vi "test Quadrature.vi"(8 "error in (no error)":errorcluster, 11 "TestCase in":refnum<class "Scan Engine cRIO System Tests.lvclass">) -> (0 "error out":errorcluster, 3 "TestCase out":refnum<class "Scan Engine cRIO System Tests.lvclass">)   [LabVIEW 2016, in "Scan Engine cRIO System Tests.lvclass"]
uses:
  Scan Engine cRIO System Tests.lvclass
  C:/Users/rzoeller/Documents/ni-official/niveristand-custom-device-testing-tools/VeriStandTestCase/VeriStandTestCase.lvclass
  <vilib>/NI Veristand/Execution/Workspace/NI VeriStand - Get Single Channel Value.vi
  <vilib>/addons/_JKI Toolkits/VI Tester/TestCase.llb/TestCase.lvclass
  <vilib>/NI VeriStand/Execution/Workspace/NI_VS Workspace ExecutionAPI.lvlib
  C:/Program Files (x86)/National Instruments/LabVIEW 2016/vi.lib/addons/_JKI Toolkits/VI Tester/TestCase.llb/TestCase.lvclass
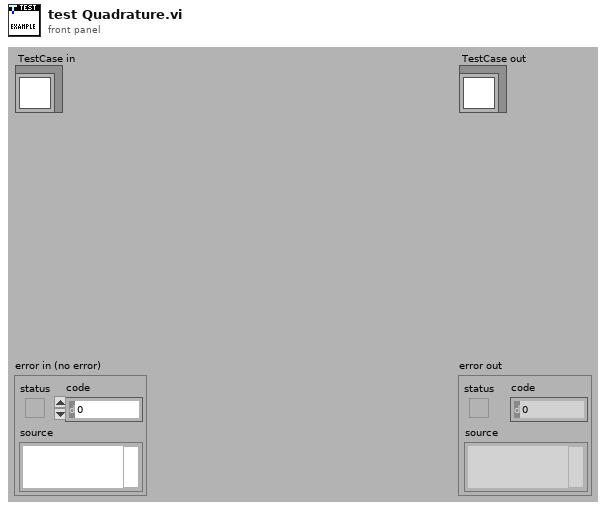
[diagram p1: front panel]
types:
  T1 = typedef "NI_VS Workspace ExecutionAPI.lvlib/WorkspaceAPI.ctl" = refnum<k24>
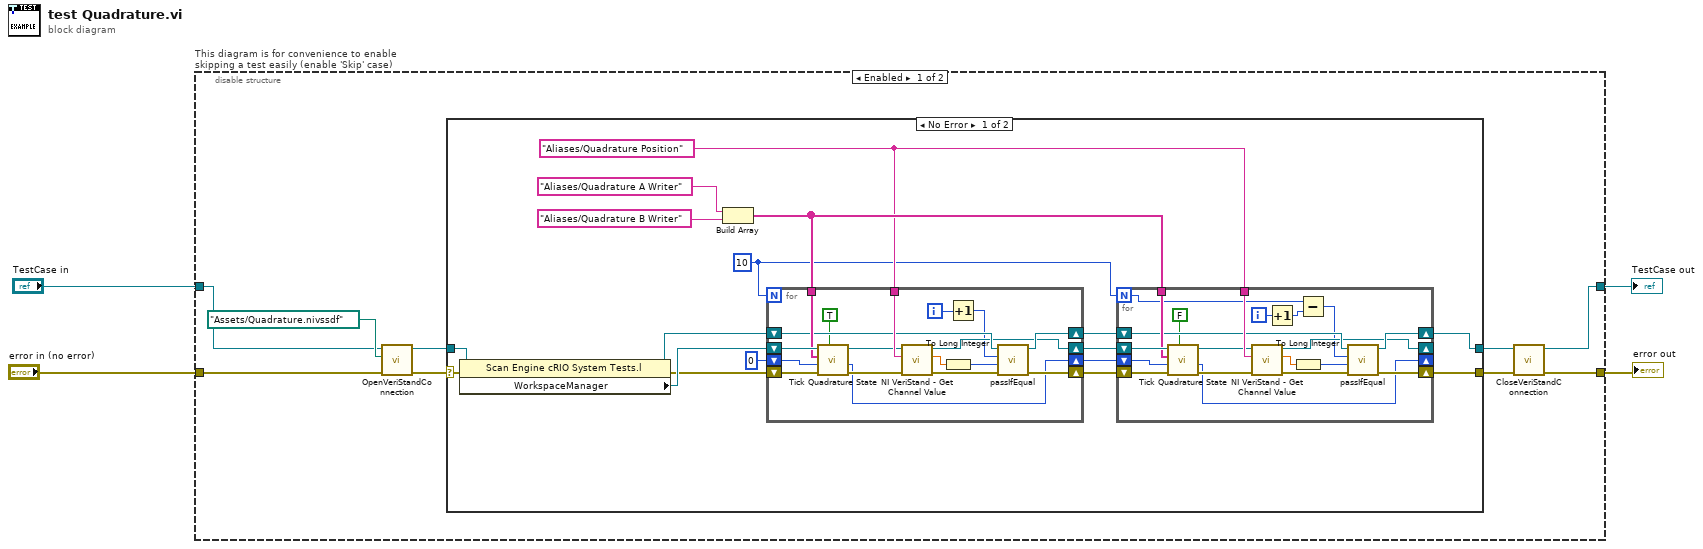
[diagram p0: block diagram]
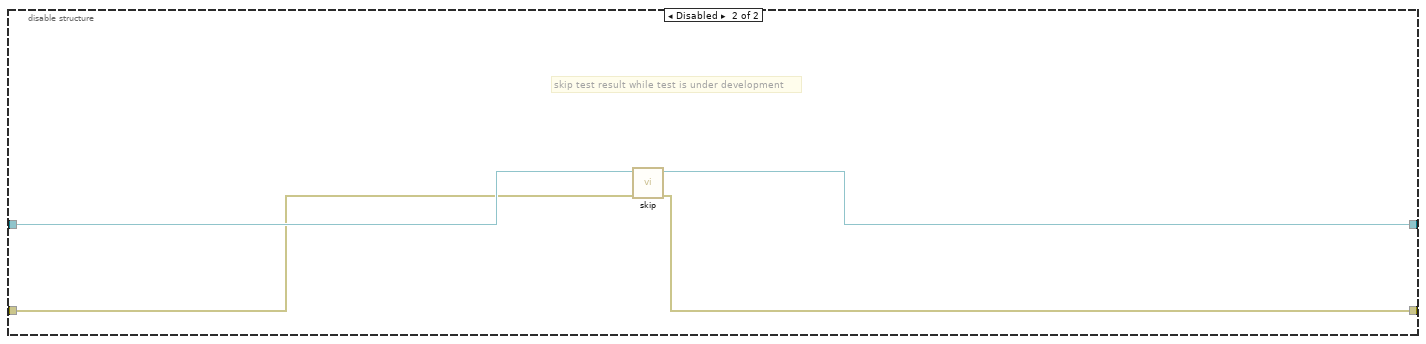
[diagram p3: hidden frame]
diagram:
  n1 = disable-structure "This diagram is for convenience to enable skipping a test easily (enable 'Skip' case)" shown="Enabled" {
    disable-tunnel: "TestCase in" -> [w9 w74]
    disable-tunnel: [w6 w72] -> w1
    disable-tunnel: [w7 w73] -> w3
    disable-tunnel: "error in (no error)" -> [w11 w71]
    frame Enabled {
      n2 = call-dynamic "OpenVeriStandConnection.vi"("error in (no error)"=w11, "System Definition File"=path "Assets/Quadrature.nivssdf", "VeriStand Test Case in"=w9) -> ("error out"=w12:errorcluster, "VeriStand Test Case out"=w10:refnum<class "Scan Engine cRIO System Tests.lvclass">)  [unwired: 7 in]
      n3 = case shown="No Error" w12 {
        selector: w12 -> [w30 w70]
        tunnel: [w15 w70] -> w8
        tunnel: [w14 w69] -> w5
        tunnel: w10 -> [w29 w69]
        frame No Error {
          w18 = 10
          w21 = "Aliases/Quadrature Position" ("Channel")
          n4 = property class="Scan Engine cRIO System Tests.l"(reference=w29, error in=w30) -> (reference out=w24:refnum<class "Scan Engine cRIO System Tests.lvclass">, error out=w27:errorcluster, "WorkspaceManager"=w28:T1)
          n5 = Build Array("Aliases/Quadrature A Writer" ("Channel"), "Aliases/Quadrature B Writer" ("Channel")) -> (w22:string[])
          n6 = for {
            N: w18 -> [_]
            tunnel: w21 -> [w68]
            tunnel: w22 -> [w59]
            shift-right: [w66] -> w19
            shift-left: w27 -> [w61]
            shift-right: [w65] -> w20
            shift-left: w24 -> [w58]
            shift-right: [w56] -> w17
            shift-left: 0 ("New State") -> [w57]
            shift-right: [w55] -> w16
            shift-left: w28 -> [w62]
            i -> [w53]
            n7 = call "Tick Quadrature State.vi"("Forward? (T)"=TRUE, "error in (no error)"=w61, "Current State"=w57, "Channels"=w59, "WorkspaceManager in"=w62) -> ("error out"=w60:errorcluster, "New State"=w56:i32, "WorkspaceManager out"=w63:T1)  [unwired: 4 in]
            n8 = call-poly <vilib>:"NI VeriStand - Get Channel Value.vi"("error in (no error)"=w60, "Channel"=w68, "WorkspaceManager in"=w63) -> ("error out"=w67:errorcluster, "Value"=w64:dbl, "WorkspaceManager out"=w55:T1)  [unwired: 6 in]
            n9 = To Long Integer(number=w64) -> (32bit integer=w52:i32)
            n10 = Increment(x=w53) -> (x+1=w51:i32)
            n11 = call-dynamic "passIfEqual.vi"("error in (no error)"=w67, "y"=w52, "x"=w51, "TestCase in"=w58) -> ("error out"=w66:errorcluster, "TestCase out"=w65:refnum<class "Scan Engine cRIO System Tests.lvclass">)  [unwired: 6 in]
          }
          n12 = for {
            N: w18 -> [w34]
            tunnel: w21 -> [w50]
            tunnel: w22 -> [w41]
            shift-right: [w48] -> w15
            shift-left: w19 -> [w43]
            shift-right: [w47] -> w14
            shift-left: w20 -> [w40]
            shift-right: [w38] -> _
            shift-left: w17 -> [w39]
            shift-right: [w37] -> _
            shift-left: w16 -> [w44]
            i -> [w33]
            n13 = call "Tick Quadrature State.vi"("Forward? (T)"=FALSE, "error in (no error)"=w43, "Current State"=w39, "Channels"=w41, "WorkspaceManager in"=w44) -> ("error out"=w42:errorcluster, "New State"=w38:i32, "WorkspaceManager out"=w45:T1)  [unwired: 4 in]
            n14 = call-poly <vilib>:"NI VeriStand - Get Channel Value.vi"("error in (no error)"=w42, "Channel"=w50, "WorkspaceManager in"=w45) -> ("error out"=w49:errorcluster, "Value"=w46:dbl, "WorkspaceManager out"=w37:T1)  [unwired: 6 in]
            n15 = Increment(x=w33) -> (x+1=w32:i32)
            n16 = To Long Integer(number=w46) -> (32bit integer=w35:i32)
            n17 = Subtract(x=w34, y=w32) -> (x-y=w31:i32)
            n18 = call-dynamic "passIfEqual.vi"("error in (no error)"=w49, "y"=w35, "x"=w31, "TestCase in"=w40) -> ("error out"=w48:errorcluster, "TestCase out"=w47:refnum<class "Scan Engine cRIO System Tests.lvclass">)  [unwired: 6 in]
          }
        }
        frame Error {
        }
      }
      n19 = call-dynamic "CloseVeriStandConnection.vi"("error in (no error)"=w8, "VeriStand Test Case in"=w5) -> ("error out"=w7:errorcluster, "VeriStand Test Case out"=w6:refnum<class "Scan Engine cRIO System Tests.lvclass">)  [unwired: 8 in]
    }
    frame Disabled {
      # "skip test result while test is under development"
      n20 = call <vilib>:"skip.vi"("error in (no error)"=w71, "TestCase in"=w74) -> ("error out"=w73:errorcluster, "TestCase out"=w72:refnum<class "Scan Engine cRIO System Tests.lvclass">)  [unwired: 8 in]
    }
  }
  "error out" <- w3
  "TestCase out" <- w1
